vi "Verticle Angles.vi"(10 "Data Points":T2(array[cluster])) -> (2 "New Data Points":T1(array[cluster]))   [LabVIEW 2017]
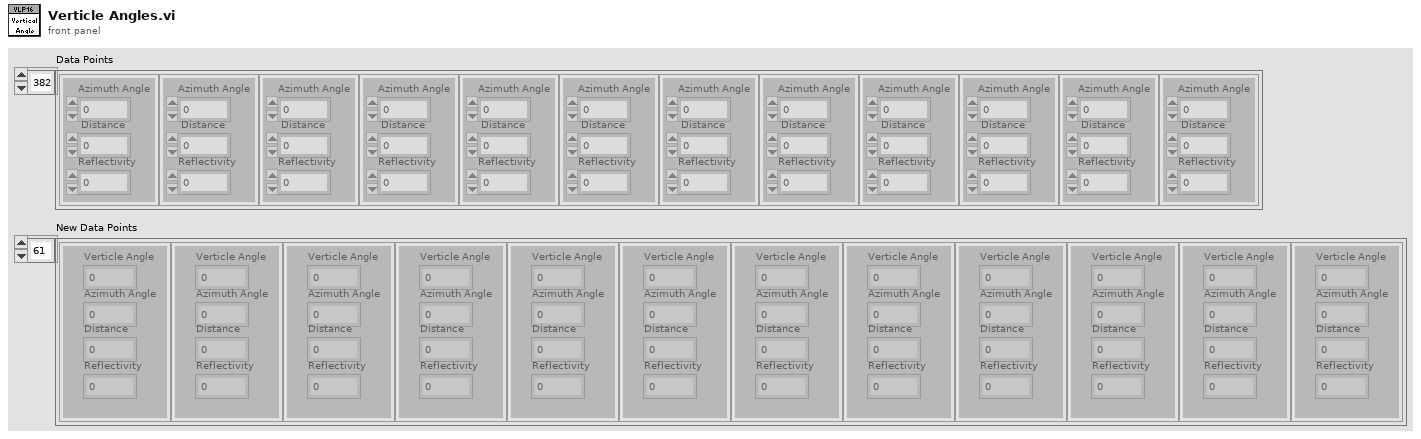
[diagram p1: front panel]
types:
  T1 = cluster{"Verticle Angle":dbl, "Azimuth Angle":dbl, "Distance":dbl, "Reflectivity":dbl}[]
  T2 = cluster{"Azimuth Angle":dbl, " Distance":dbl, "Reflectivity":dbl}[]
  T3 = cluster{dbl, "Azimuth Angle":dbl, " Distance":dbl, "Reflectivity":dbl}
  T4 = cluster{dbl, "Azimuth Angle":dbl, " Distance":dbl, "Reflectivity":dbl}[]
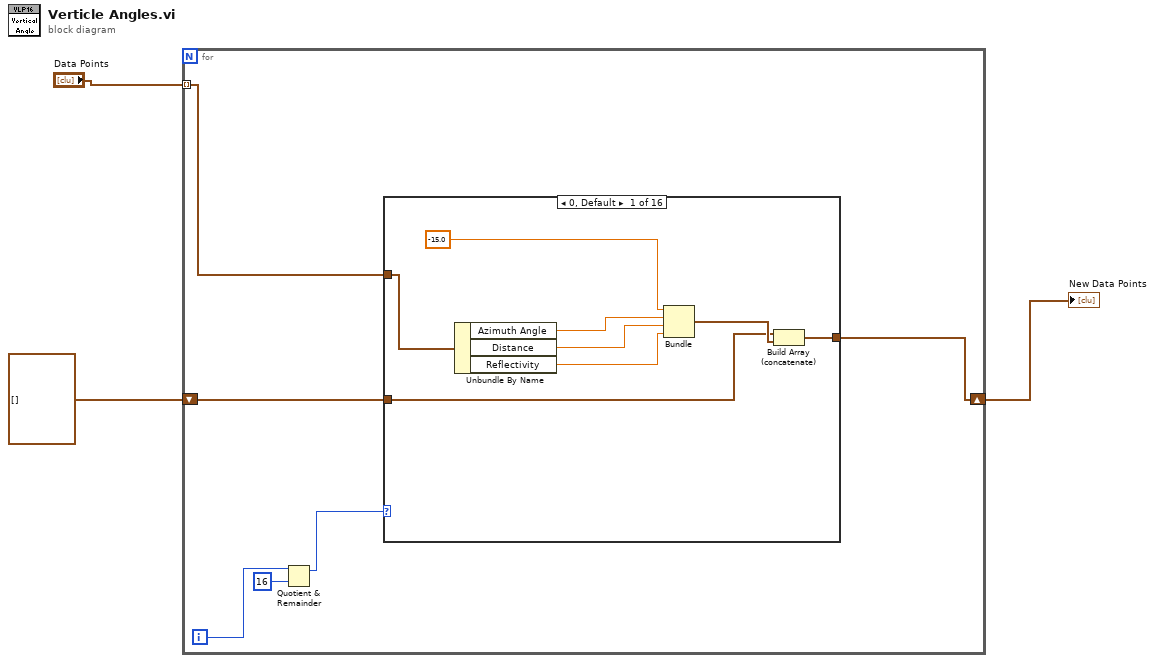
[diagram p0: block diagram]
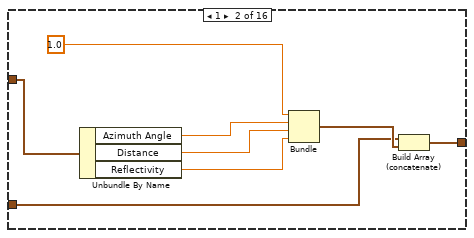
[diagram p2: hidden frame]
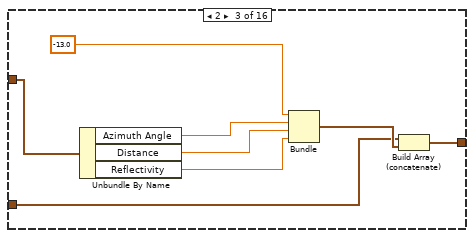
[diagram p3: hidden frame]
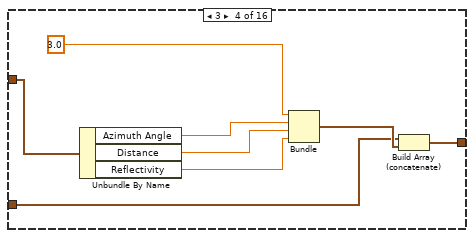
[diagram p4: hidden frame]
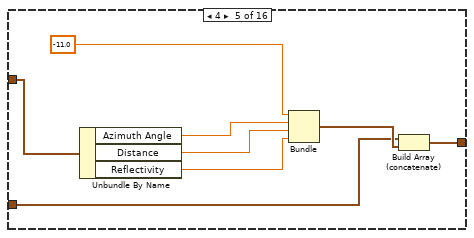
[diagram p5: hidden frame]
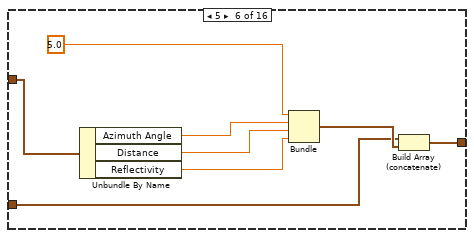
[diagram p6: hidden frame]
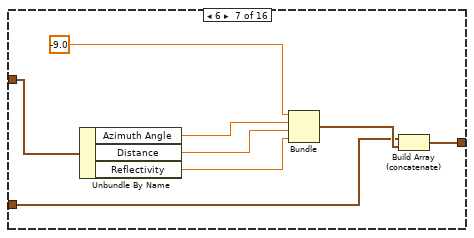
[diagram p7: hidden frame]
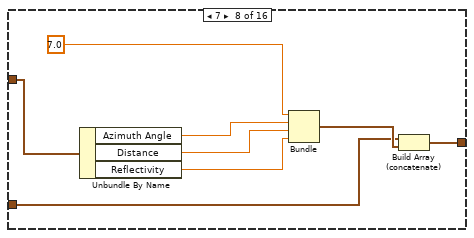
[diagram p8: hidden frame]
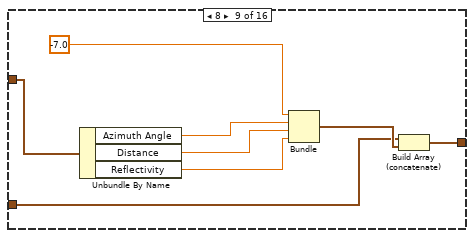
[diagram p9: hidden frame]
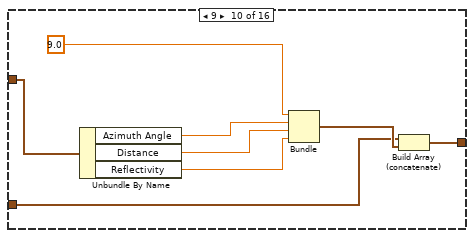
[diagram p10: hidden frame]
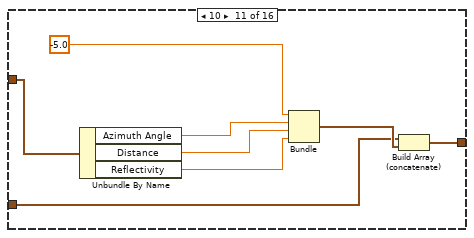
[diagram p11: hidden frame]
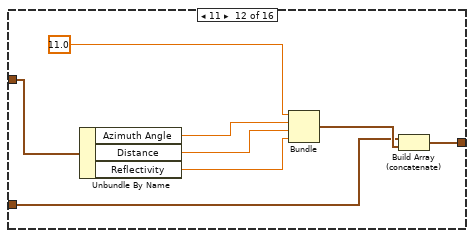
[diagram p12: hidden frame]
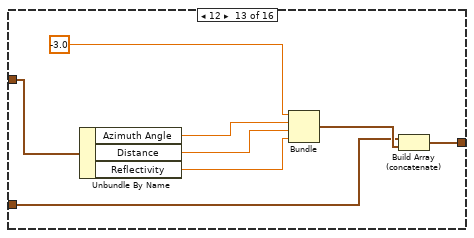
[diagram p13: hidden frame]
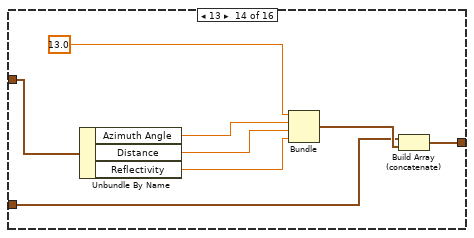
[diagram p14: hidden frame]
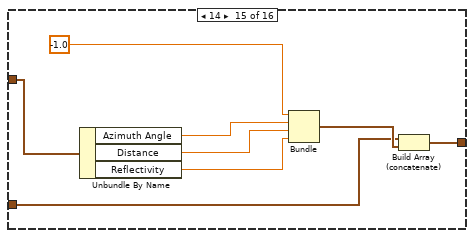
[diagram p15: hidden frame]
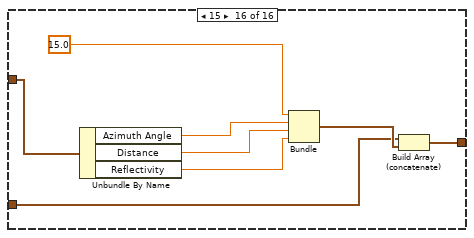
[diagram p16: hidden frame]
diagram:
  n1 = for {
    tunnel: "Data Points" -> [w9] mode=indexing
    shift-right: [w7] -> w1
    shift-left: cluster{dbl, dbl, dbl, dbl}[] [] -> [w8]
    i -> [w6]
    n2 = Quotient & Remainder(x=w6, y=16) -> (x-y*floor(x/y)=w4:i32)  [unwired: 1 out]
    n3 = case shown="0, Default" w4 {
      tunnel: w9 -> [w17 w25 w33 w41 w49 w57 w65 w73 w81 w89 w97 w105 w113 w121 w129 w137]
      tunnel: w8 -> [w11 w19 w27 w35 w43 w51 w59 w67 w75 w83 w91 w99 w107 w115 w123 w131]
      tunnel: [w10 w18 w26 w34 w42 w50 w58 w66 w74 w82 w90 w98 w106 w114 w122 w130] -> w7
      frame 0, Default {
        n4 = Unbundle By Name(w17) -> ("Azimuth Angle"=w15:dbl, "Distance"=w14:dbl, "Reflectivity"=w13:dbl)
        n5 = Bundle(-15.0, "Azimuth Angle"=w15, "Distance"=w14, "Reflectivity"=w13) -> (w12:T3)  [unwired: 1 in]
        n6 = Build Array (concatenate)(w11, w12) -> (w10:T4)
      }
      frame 1 {
        n7 = Unbundle By Name(w25) -> ("Azimuth Angle"=w23:dbl, "Distance"=w22:dbl, "Reflectivity"=w21:dbl)
        n8 = Bundle(1.0, "Azimuth Angle"=w23, "Distance"=w22, "Reflectivity"=w21) -> (w20:T3)  [unwired: 1 in]
        n9 = Build Array (concatenate)(w19, w20) -> (w18:T4)
      }
      frame 2 {
        n10 = Unbundle By Name(w33) -> ("Azimuth Angle"=w31:dbl, "Distance"=w30:dbl, "Reflectivity"=w29:dbl)
        n11 = Bundle(-13.0, "Azimuth Angle"=w31, "Distance"=w30, "Reflectivity"=w29) -> (w28:T3)  [unwired: 1 in]
        n12 = Build Array (concatenate)(w27, w28) -> (w26:T4)
      }
      frame 3 {
        n13 = Unbundle By Name(w41) -> ("Azimuth Angle"=w39:dbl, "Distance"=w38:dbl, "Reflectivity"=w37:dbl)
        n14 = Bundle(3.0, "Azimuth Angle"=w39, "Distance"=w38, "Reflectivity"=w37) -> (w36:T3)  [unwired: 1 in]
        n15 = Build Array (concatenate)(w35, w36) -> (w34:T4)
      }
      frame 4 {
        n16 = Unbundle By Name(w49) -> ("Azimuth Angle"=w47:dbl, "Distance"=w46:dbl, "Reflectivity"=w45:dbl)
        n17 = Bundle(-11.0, "Azimuth Angle"=w47, "Distance"=w46, "Reflectivity"=w45) -> (w44:T3)  [unwired: 1 in]
        n18 = Build Array (concatenate)(w43, w44) -> (w42:T4)
      }
      frame 5 {
        n19 = Unbundle By Name(w57) -> ("Azimuth Angle"=w55:dbl, "Distance"=w54:dbl, "Reflectivity"=w53:dbl)
        n20 = Bundle(5.0, "Azimuth Angle"=w55, "Distance"=w54, "Reflectivity"=w53) -> (w52:T3)  [unwired: 1 in]
        n21 = Build Array (concatenate)(w51, w52) -> (w50:T4)
      }
      frame 6 {
        n22 = Unbundle By Name(w65) -> ("Azimuth Angle"=w63:dbl, "Distance"=w62:dbl, "Reflectivity"=w61:dbl)
        n23 = Bundle(-9.0, "Azimuth Angle"=w63, "Distance"=w62, "Reflectivity"=w61) -> (w60:T3)  [unwired: 1 in]
        n24 = Build Array (concatenate)(w59, w60) -> (w58:T4)
      }
      frame 7 {
        n25 = Unbundle By Name(w73) -> ("Azimuth Angle"=w71:dbl, "Distance"=w70:dbl, "Reflectivity"=w69:dbl)
        n26 = Bundle(7.0, "Azimuth Angle"=w71, "Distance"=w70, "Reflectivity"=w69) -> (w68:T3)  [unwired: 1 in]
        n27 = Build Array (concatenate)(w67, w68) -> (w66:T4)
      }
      frame 8 {
        n28 = Unbundle By Name(w81) -> ("Azimuth Angle"=w79:dbl, "Distance"=w78:dbl, "Reflectivity"=w77:dbl)
        n29 = Bundle(-7.0, "Azimuth Angle"=w79, "Distance"=w78, "Reflectivity"=w77) -> (w76:T3)  [unwired: 1 in]
        n30 = Build Array (concatenate)(w75, w76) -> (w74:T4)
      }
      frame 9 {
        n31 = Unbundle By Name(w89) -> ("Azimuth Angle"=w87:dbl, "Distance"=w86:dbl, "Reflectivity"=w85:dbl)
        n32 = Bundle(9.0, "Azimuth Angle"=w87, "Distance"=w86, "Reflectivity"=w85) -> (w84:T3)  [unwired: 1 in]
        n33 = Build Array (concatenate)(w83, w84) -> (w82:T4)
      }
      frame 10 {
        n34 = Unbundle By Name(w97) -> ("Azimuth Angle"=w95:dbl, "Distance"=w94:dbl, "Reflectivity"=w93:dbl)
        n35 = Bundle(-5.0, "Azimuth Angle"=w95, "Distance"=w94, "Reflectivity"=w93) -> (w92:T3)  [unwired: 1 in]
        n36 = Build Array (concatenate)(w91, w92) -> (w90:T4)
      }
      frame 11 {
        n37 = Unbundle By Name(w105) -> ("Azimuth Angle"=w103:dbl, "Distance"=w102:dbl, "Reflectivity"=w101:dbl)
        n38 = Bundle(11.0, "Azimuth Angle"=w103, "Distance"=w102, "Reflectivity"=w101) -> (w100:T3)  [unwired: 1 in]
        n39 = Build Array (concatenate)(w99, w100) -> (w98:T4)
      }
      frame 12 {
        n40 = Unbundle By Name(w113) -> ("Azimuth Angle"=w111:dbl, "Distance"=w110:dbl, "Reflectivity"=w109:dbl)
        n41 = Bundle(-3.0, "Azimuth Angle"=w111, "Distance"=w110, "Reflectivity"=w109) -> (w108:T3)  [unwired: 1 in]
        n42 = Build Array (concatenate)(w107, w108) -> (w106:T4)
      }
      frame 13 {
        n43 = Unbundle By Name(w121) -> ("Azimuth Angle"=w119:dbl, "Distance"=w118:dbl, "Reflectivity"=w117:dbl)
        n44 = Bundle(13.0, "Azimuth Angle"=w119, "Distance"=w118, "Reflectivity"=w117) -> (w116:T3)  [unwired: 1 in]
        n45 = Build Array (concatenate)(w115, w116) -> (w114:T4)
      }
      frame 14 {
        n46 = Unbundle By Name(w129) -> ("Azimuth Angle"=w127:dbl, "Distance"=w126:dbl, "Reflectivity"=w125:dbl)
        n47 = Bundle(-1.0, "Azimuth Angle"=w127, "Distance"=w126, "Reflectivity"=w125) -> (w124:T3)  [unwired: 1 in]
        n48 = Build Array (concatenate)(w123, w124) -> (w122:T4)
      }
      frame 15 {
        n49 = Unbundle By Name(w137) -> ("Azimuth Angle"=w135:dbl, "Distance"=w134:dbl, "Reflectivity"=w133:dbl)
        n50 = Bundle(15.0, "Azimuth Angle"=w135, "Distance"=w134, "Reflectivity"=w133) -> (w132:T3)  [unwired: 1 in]
        n51 = Build Array (concatenate)(w131, w132) -> (w130:T4)
      }
    }
  }
  "New Data Points" <- w1
